vi "UpdateStatus.vi"(8 "error in (no error)":errorcluster, 10 "Status":string, 11 "Comics in":refnum<class "Comics.lvclass">) -> (0 "error out":errorcluster, 3 "Comics out":refnum<class "Comics.lvclass">)   [LabVIEW 2022 SP3, in "Comics.lvclass"]
uses:
  Comics.lvclass
  Comics.lvclass/Comics.ctl
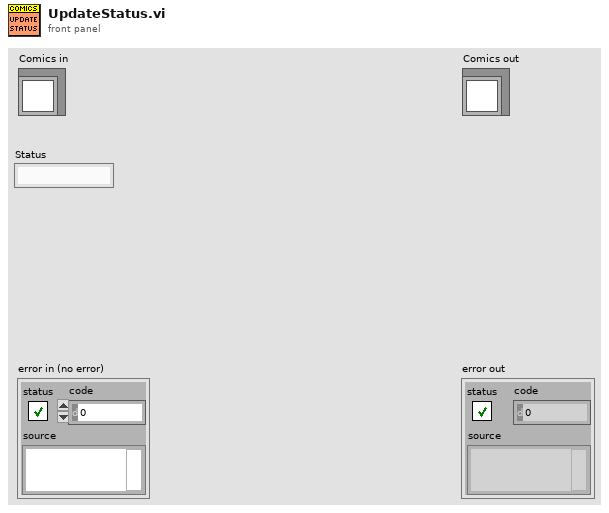
[diagram p1: front panel]
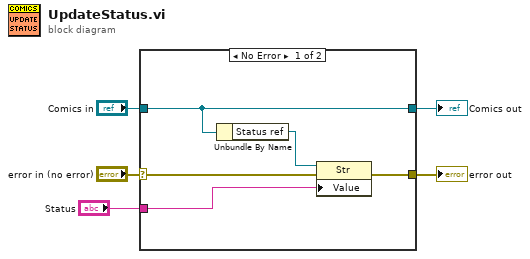
[diagram p0: block diagram]
diagram:
  n1 = case shown="No Error" "error in (no error)" {
    selector: "error in (no error)" -> [w9 w12]
    tunnel: [w8 w12] -> w4
    tunnel: [w10 w11] -> w2
    tunnel: "Comics in" -> [w10 w11]
    tunnel: "Status" -> [w6 _]
    frame No Error {
      n2 = Unbundle By Name(w10) -> ("Status ref"=w7:refnum<vi>)
      n3 = property class="Str"(reference=w7, error in=w9, "Value"=w6) -> (error out=w8:errorcluster)  [unwired: 1 out]
    }
    frame Error {
    }
  }
  "error out" <- w4
  "Comics out" <- w2
